vi "getNumOfFieldInQwgt.vi"(8 "error in (no error)":errorcluster, 11 "OptCtrl in":refnum<class "OptCtrl.lvclass">) -> (0 "error out":errorcluster, 2 "Num of Field":i32, 3 "OptCtrl out":refnum<class "OptCtrl.lvclass">)   [LabVIEW 2016, in "OptCtrl.lvclass"]
doc: "Get the number of field in the image quality weighting ratio."
uses:
  OptCtrl.lvclass
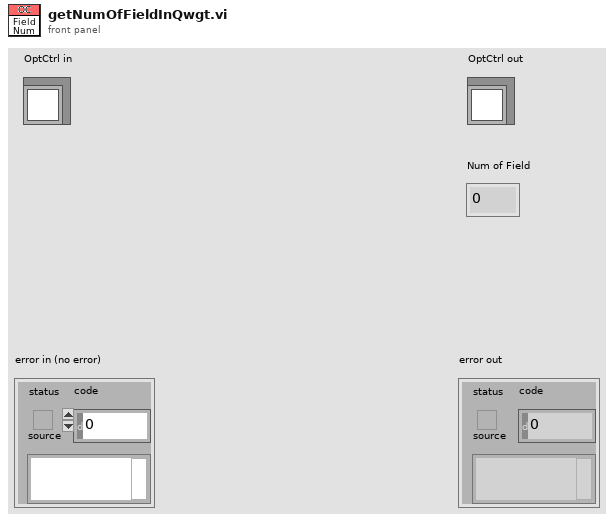
[diagram p1: front panel]
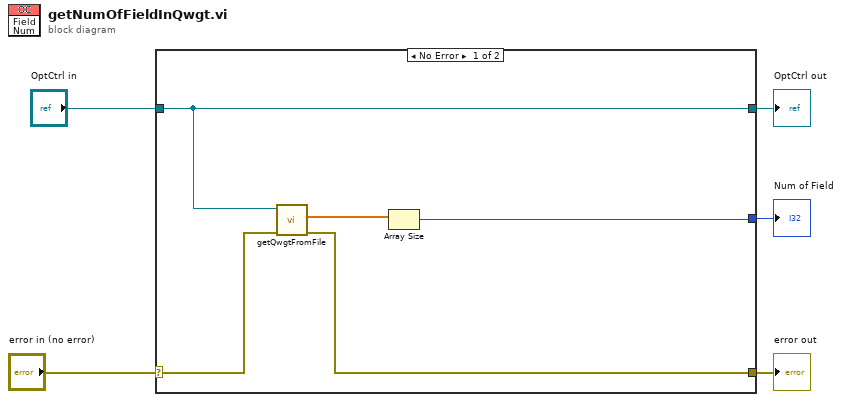
[diagram p0: block diagram]
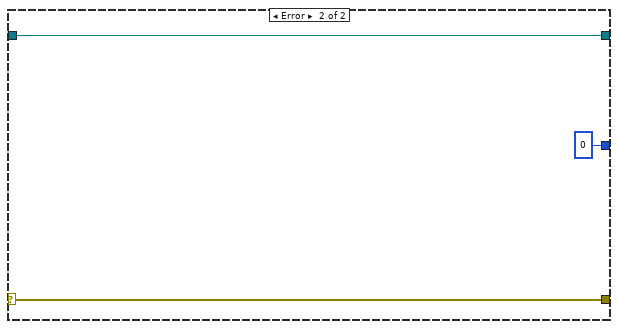
[diagram p2: hidden frame]
diagram:
  n1 = case shown="No Error" "error in (no error)" {
    selector: "error in (no error)" -> [w9 w13]
    tunnel: [w8 w13] -> w4
    tunnel: [w10 w12] -> w2
    tunnel: "OptCtrl in" -> [w10 w12]
    tunnel: [w6 0] -> w1
    frame No Error {
      n2 = call "getQwgtFromFile.vi"("error in (no error)"=w9, "OptCtrl in"=w10) -> ("error out"=w8:errorcluster, "Wgt of Q"=w7:dbl[])  [unwired: 7 in, 1 out]
      n3 = Array Size(array=w7) -> (size(s)=w6:i32)
    }
    frame Error {
    }
  }
  "error out" <- w4
  "OptCtrl out" <- w2
  "Num of Field" <- w1
